vi "free enumerate devices.vi"(8 "error in (no error)":errorcluster, 11 "device_enumeration":u64) -> (0 "error out":errorcluster, 3 "function return":i32)   [LabVIEW 2017, in "libximc.lvlib"]
doc: "result_t XIMC_API free_enumerate_devices(device_enumeration_t device_enumeration);"
uses:
  libximc.lvlib
  libximc.dll
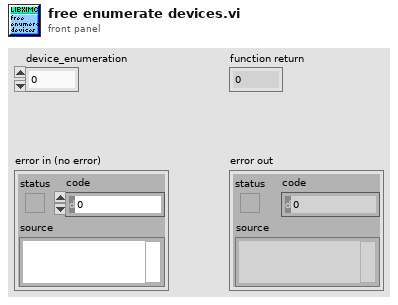
[diagram p1: front panel]
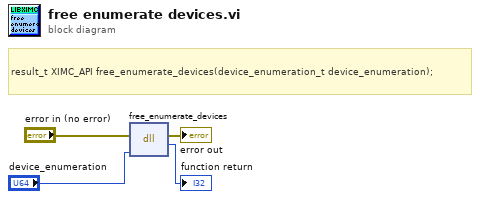
[diagram p0: block diagram]
diagram:
  # "result_t XIMC_API free_enumerate_devices(device_enumeration_t device_enumeration);"
  n1 = dll-call lib="C:/Technology Lab/NI-2010/Drivers/Standa-Motorized Iris Diaphragm/Archive/labview-2.9.12-Labview_12.0/labview-2.9.12-Labview_12.0/ximcLVx64/libximc.*" fn="free_enumerate_devices"(error in="error in (no error)", "device_enumeration"="device_enumeration") -> (error out=→"error out":errorcluster, →"function return":i32)  [unwired: 3 in, 1 out]
